vi "DVAJ common.vi"(8 "J":dbl, 9 "A":dbl, 10 "V":dbl, 11 "D":dbl) -> (2 "Amax":dbl, 3 "Vmax":dbl)   [LabVIEW 2019]
panel:
  out "x > y?":bool
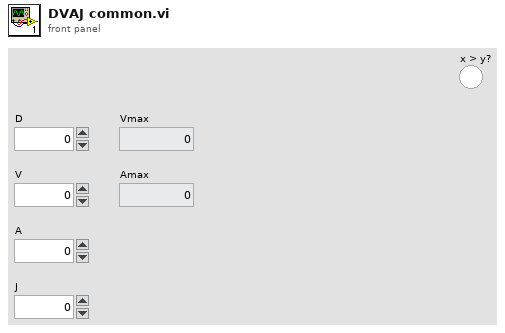
[diagram p1: front panel]
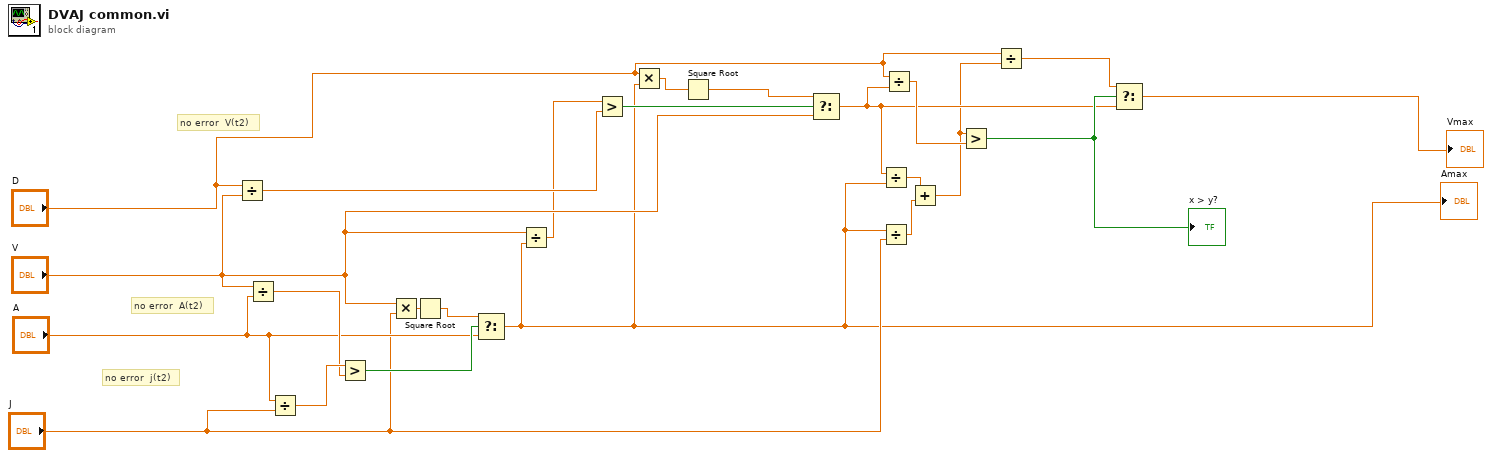
[diagram p0: block diagram]
diagram:
  # "no error  j(t2)"
  # "no error  A(t2)"
  # "no error  V(t2)"
  n1 = Divide(x="D", y="V") -> (x/y=w21:dbl)
  n2 = Divide(x="V", y="A") -> (x/y=w18:dbl)
  n3 = Divide(x="A", y="J") -> (x/y=w19:dbl)
  n4 = Greater?(x=w19, y=w18) -> (0:w22:bool)
  n5 = Multiply(x="V", y="J") -> (x*y=w12:dbl)
  n6 = Square Root(x=w12) -> (sqrt(x)=w23:dbl)
  n7 = Select(t=w23, s=w22, f="A") -> (s? t:f=w5:dbl)
  "Amax" <- w5
  n8 = Divide(x="V", y=w5) -> (x/y=w13:dbl)
  n9 = Greater?(x=w13, y=w21) -> (0:w14:bool)
  n10 = Multiply(x="D", y=w5) -> (x*y=w16:dbl)
  n11 = Square Root(x=w16) -> (sqrt(x)=w15:dbl)
  n12 = Select(t=w15, s=w14, f="V") -> (s? t:f=w4:dbl)
  n13 = Divide(x=w4, y=w5) -> (x/y=w8:dbl)
  n14 = Divide(x=w5, y="J") -> (x/y=w9:dbl)
  n15 = Divide(x="D", y=w4) -> (x/y=w11:dbl)
  n16 = Add(x=w8, y=w9) -> (x+y=w2:dbl)
  n17 = Greater?(x=w2, y=w11) -> (0:w6:bool)
  "x > y?" <- w6
  n18 = Divide(x="D", y=w2) -> (x/y=w1:dbl)
  n19 = Select(t=w1, s=w6, f=w4) -> (s? t:f=→"Vmax":dbl)
